vi "Save to History File.vi"(8 "error in (no error)":errorcluster, 10 "Records":T1[](array[typedef]), 11 "Data Manager in":refnum<class "Data Manager.lvclass">) -> (0 "error out":errorcluster, 3 "Data Manager out":refnum<class "Data Manager.lvclass">)   [LabVIEW 2020, in "Data Manager.lvclass"]
uses:
  Data Manager.lvclass
  Strava JSON for Club Activities--cluster.ctl
  Data Manager.lvclass/Data Manager.ctl
  Name--cluster.ctl
  Profile--cluster.ctl
  <vilib>/drjdpowell/SQLite Library/SQL Statement/SQL Statement.lvclass/SQL Statement.ctl
  <vilib>/drjdpowell/SQLite Library/SQL Statement/Bind Text.vi
  <vilib>/drjdpowell/SQLite Library/SQL Statement/Bind Timestamp (Text).vi
  <vilib>/drjdpowell/SQLite Library/SQL Statement/Bind Real.vi
  <vilib>/drjdpowell/SQLite Library/SQL Statement/Bind Integer.vi
  <vilib>/drjdpowell/SQLite Library/SQL Statement/Step.vi
  <vilib>/JDP Science/JDP Science Common Utilities/Timestamp/Timestamp to Text.vi
  <vilib>/drjdpowell/SQLite Library/SQL Statement/Error Message.vi
  <vilib>/drjdpowell/SQLite Library/SQL Connection/Connection.lvclass
  <vilib>/drjdpowell/SQLite Library/SQL Statement/SQL Statement.lvclass
  <vilib>/drjdpowell/SQLite Library/Transaction Helpers/Transaction.lvlib
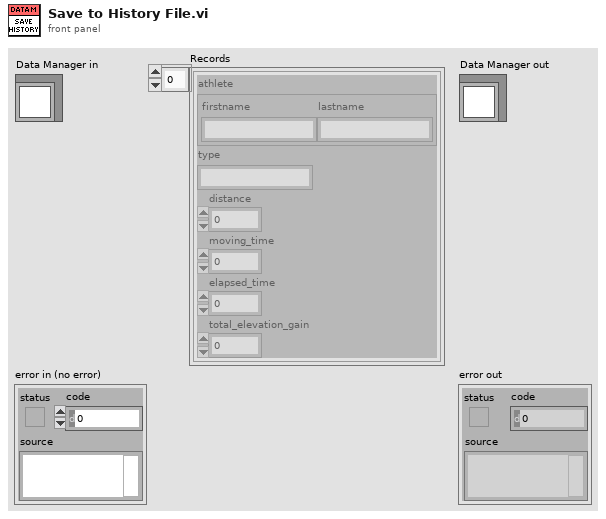
[diagram p1: front panel]
types:
  T1 = typedef "Data Manager.lvclass/Strava JSON for Club Activities--cluster.ctl" = cluster{"athlete":cluster{"firstname":string, "lastname":string}, "type":string, "distance":dbl, "moving_time":dbl, "elapsed_time":dbl, "total_elevation_gain":dbl}
  T2 = typedef "Data Manager.lvclass/Profile--cluster.ctl" = cluster{"Alias":string, "Team":string}
  T3 = typedef "Data Manager.lvclass/Name--cluster.ctl" = cluster{"First":string, "Last":string}
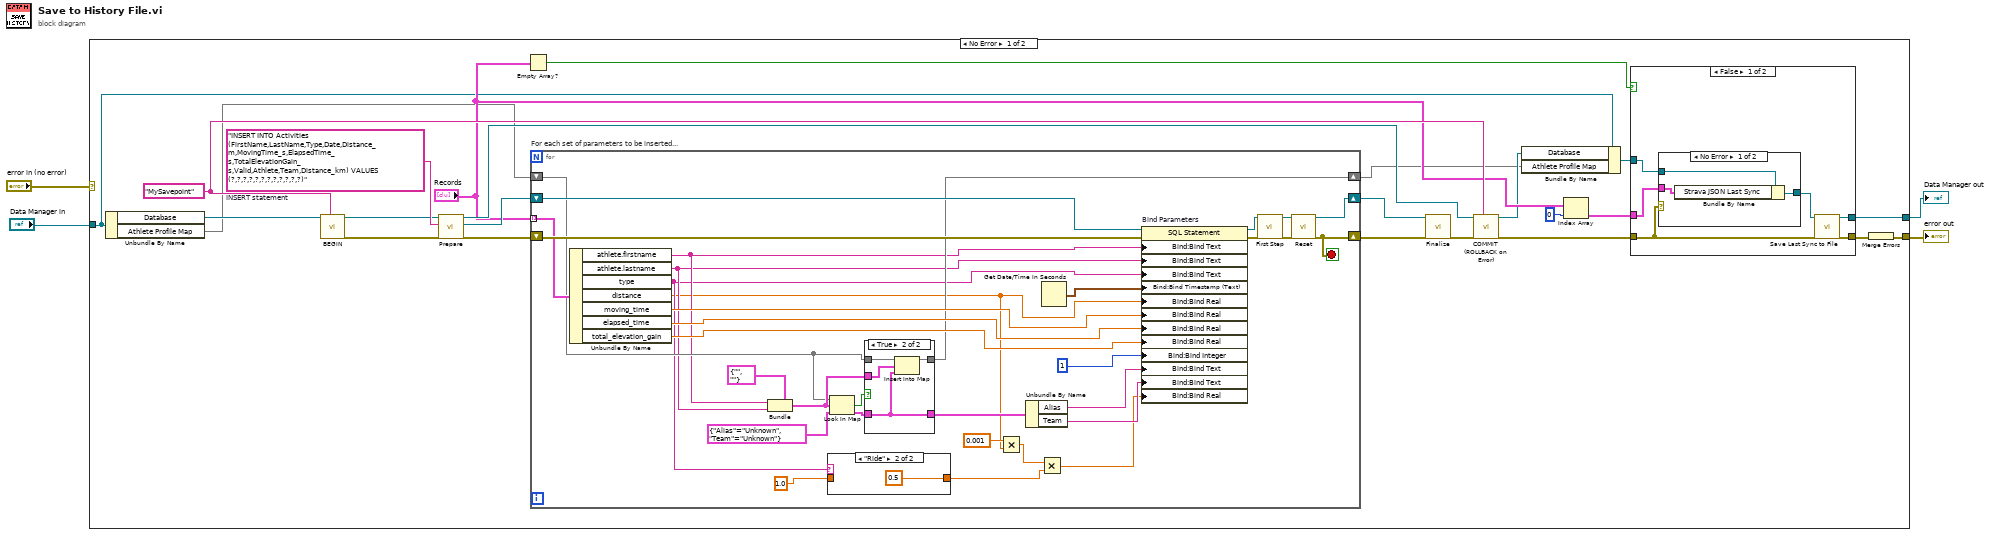
[diagram p0: block diagram]
diagram:
  n1 = case shown="No Error" "error in (no error)" {
    selector: "error in (no error)" -> [_ w83]
    tunnel: [w28 w83] -> w3
    tunnel: [w27 w82] -> w1
    tunnel: "Data Manager in" -> [w9 w82]
    frame No Error {
      w20 = "MySavepoint" ("Savepoint name")
      w16 = "INSERT INTO Activities (FirstName,LastName,Type,Date,Distance_m,MovingTime_s,ElapsedTime_s,TotalElevationGain_s,Valid,Athlete,Team,Distance_km) VALUES (?,?,?,?,?,?,?,?,?,?,?,?)"  # INSERT statement
      n2 = Unbundle By Name(w9) -> ("Database"=w10:refnum<class "Connection.lvclass">, "Athlete Profile Map"=w6:map{T3, T2})
      n3 = call <vilib>:"BEGIN.vi"("Savepoint name"=w20, "SQLite Connection in"=w10) -> ("error out"=w19:errorcluster, "SQLite Connection"=w12:refnum<class "Connection.lvclass">)  [unwired: 8 in]
      n4 = call <vilib>:"Prepare.vi"("error in (no error)"=w19, "SQL"=w16, "SQLite Connection in"=w12) -> ("error out"=w15:errorcluster, "SQL Statement"=w14:refnum<class "SQL Statement.lvclass">, "SQLite Connection"=w21:refnum<class "Connection.lvclass">)  [unwired: 4 in, 2 out]
      n5 = Empty Array?(array="Records") -> (empty?=w23:bool)
      n6 = for "For each set of parameters to be inserted..." {
        shift-right: [w55] -> w17
        shift-left: w14 -> [w61]
        shift-right: [w54] -> w18
        shift-left: w15 -> [w58]
        tunnel: "Records" -> [w53] mode=indexing
        shift-right: [w40] -> w5
        shift-left: w6 -> [w42]
        stop <- w54 stop-if-true
        n7 = Unbundle By Name(w53) -> ("athlete.firstname"=w37:string, "athlete.lastname"=w36:string, "type"=w35:string, "distance"=w32:dbl, "moving_time"=w51:dbl, "elapsed_time"=w50:dbl, "total_elevation_gain"=w49:dbl)
        n8 = Bundle(cluster=T3 {"First"="", "Last"=""} ("Name"), "First"=w37, "Last"=w36) -> (w46:T3)
        n9 = case shown="\"Ride\"" w35 {
          tunnel: [w62 0.5] -> w31
          tunnel: 1.0 -> [w62 _]
          frame "False", Default {
          }
          frame "Ride" {
          }
        }
        n10 = Look In Map(map=w42, key=w46, default value=T2 {"Alias"="Unknown", "Team"="Unknown"}) -> (key not found?=w41:bool, value=w45:T2)
        n11 = case shown="True" w41 {
          tunnel: w42 -> [w65 w69]
          tunnel: [w65 w68] -> w40
          tunnel: w45 -> [w64 w66]
          tunnel: w46 -> [_ w67]
          tunnel: [w64 w66] -> w47
          frame False {
          }
          frame True {
            n12 = Insert Into Map(map in=w69, key=w67, value=w66) -> (map out=w68:map{T3, T2})  [unwired: 2 out]
          }
        }
        n13 = Multiply(x=0.001, y=w32) -> (x*y=w33:dbl)
        n14 = Unbundle By Name(w47) -> ("Alias"=w39:string, "Team"=w38:string)
        n15 = Multiply(x=w33, y=w31) -> (x*y=w29:dbl)
        n16 = Get Date/Time In Seconds() -> (seconds since 1Jan1904=w52:timestamp)
        n17 = property on="Bind Parameters" class="SQL Statement"(reference=w61, error in=w58, "Bind:Bind Text"=w37, "Bind:Bind Text"=w36, "Bind:Bind Text"=w35, "Bind:Bind Timestamp (Text)"=w52, "Bind:Bind Real"=w32, "Bind:Bind Real"=w51, "Bind:Bind Real"=w50, "Bind:Bind Real"=w49, "Bind:Bind Integer"=i64 1 ("Bind:Integer"), "Bind:Bind Text"=w39, "Bind:Bind Text"=w38, "Bind:Bind Real"=w29) -> (reference out=w60:refnum<class "SQL Statement.lvclass">, error out=w59:errorcluster)
        n18 = call <vilib>:"First Step.vi"("error in (no error)"=w59, "SQL Statement in"=w60) -> ("error out"=w57:errorcluster, "SQL Statement"=w56:refnum<class "SQL Statement.lvclass">)  [unwired: 7 in, 1 out]
        n19 = call <vilib>:"Reset.vi"("error in (no error)"=w57, "SQL Statement in"=w56) -> ("error out"=w54:errorcluster, "SQL Statement"=w55:refnum<class "SQL Statement.lvclass">)  [unwired: 8 in]
      }
      n20 = call <vilib>:"Finalize.vi"("error in (no error)"=w18, "SQL Statement in"=w17) -> ("error out"=w22:errorcluster)  [unwired: 9 in]
      n21 = call <vilib>:"COMMIT (ROLLBACK on Error).vi"("Savepoint name"=w20, "error in (no error)"=w22, "SQLite Connection in"=w21) -> ("error out"=w11:errorcluster, "SQLite Connection"=w7:refnum<class "Connection.lvclass">)  [unwired: 7 in]
      n22 = Bundle By Name(cluster=w9, "Database"=w7, "Athlete Profile Map"=w5) -> (w8:refnum<class "Data Manager.lvclass">)
      n23 = Index Array(array="Records", index=0) -> (element=w25:T1)
      n24 = case shown="False" w23 {
        tunnel: w11 -> [w75 w80]
        tunnel: w8 -> [w74 w81]
        tunnel: [w72 w81] -> w27
        tunnel: [w71 w80] -> w26
        tunnel: w25 -> [w70 _]
        frame False {
          n25 = case shown="No Error" w75 {
            tunnel: w74 -> [w78 w79]
            tunnel: [w77 w79] -> w73
            tunnel: w70 -> [w76 _]
            frame No Error {
              n26 = Bundle By Name(cluster=w78, "Strava JSON Last Sync"=w76) -> (w77:refnum<class "Data Manager.lvclass">)
            }
            frame Error {
            }
          }
          n27 = call-dynamic "Save Last Sync to File.vi"("error in (no error)"=w75, "Data Manager in"=w73) -> ("error out"=w71:errorcluster, "Data Manager out"=w72:refnum<class "Data Manager.lvclass">)  [unwired: 8 in]
        }
        frame True {
        }
      }
      n28 = Merge Errors(w26) -> (w28:errorcluster)
    }
    frame Error {
    }
  }
  "error out" <- w3
  "Data Manager out" <- w1
